vi "Get SMO PGSQL Log Paths.vi"(5 "getAll Cluster":variant, 7 "Paths":string="llab_038:d000(TEST_TABLE--Temperature(Kelvin))\nllab_038:d002(TEST_TABLE--voltage 2(volts))\nllab_038:b000(TEST_TABLE--ON?())\nllab_038:v001(TEST_TABLE--sample())", 8 "error in (no error)":errorcluster, 11 "Inst.SPC in":refnum<class "Inst.SPC.lvclass">) -> (0 "error out":errorcluster, 2 "Paths":string, 3 "Inst.SPC out":refnum<class "Inst.SPC.lvclass">)   [LabVIEW 2019, in "Inst.SPC.lvclass"]
uses:
  Inst.SPC.lvclass
  Typedefs/Inst.SPC.getAll--Cluster.ctl
  <userlib>/LevyLab/Instrument Framework/Instrument Types/VSource/Instrument.VSource.lvclass
  <userlib>/LevyLab/LV-Data/LV-Data.PG/LV-Data.PGSQL.lvclass
  <userlib>/LevyLab/LV-Data/LV-Data.PG/API/Write Variable (one-row).vi
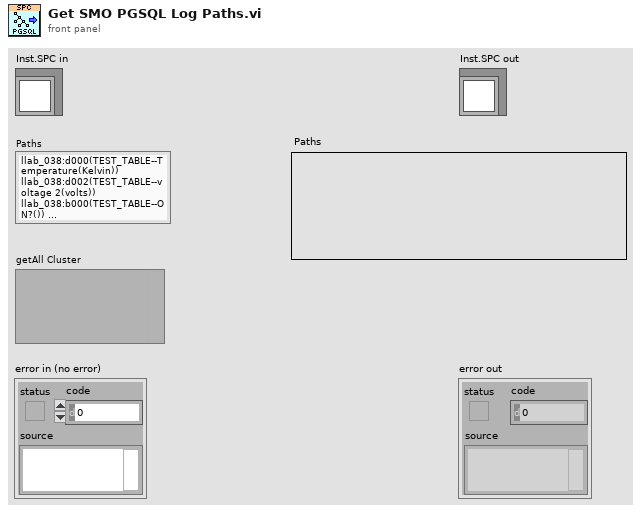
[diagram p1: front panel]
types:
  T1 = typedef "Inst.SPC.lvclass/Inst.SPC.getAll--Cluster.ctl" = cluster{"Levy 1":dbl, "Logger SMO":dbl, "SMO Boolean":bool, "SMO String":string}
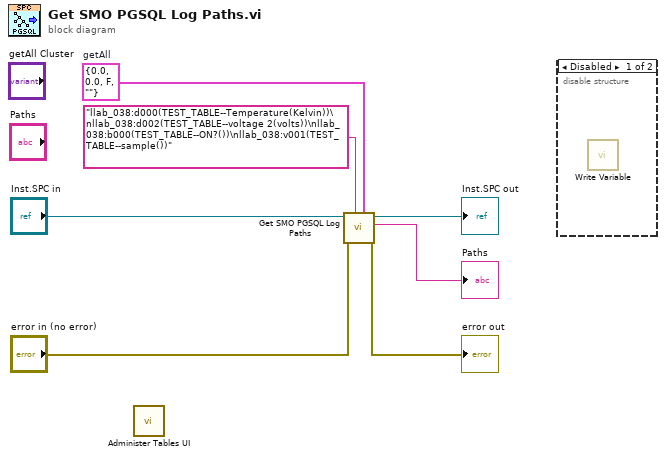
[diagram p0: block diagram]
diagram:
  w1 = T1 {"Levy 1"=0.0, "Logger SMO"=0.0, "SMO Boolean"=FALSE, "SMO String"=""}  # getAll
  n1 = call <userlib>:"Administer Tables UI.vi"() -> ()  [unwired: 12 in]
  n2 = call-parent "Get SMO PGSQL Log Paths.vi"("getAll Cluster"=w1, "Default Paths"="llab_038:d000(TEST_TABLE--Temperature(Kelvin))\nllab_038:d002(TEST_TABLE--voltage 2(volts))\nllab_038:b000(TEST_TABLE--ON?())\nllab_038:v001(TEST_TABLE--sample())" ("Paths"), "error in (no error)"="error in (no error)", "Instrument in"="Inst.SPC in") -> ("error out"=→"error out":errorcluster, "Paths"=→"Paths":string, "Instrument out"=→"Inst.SPC out":refnum<class "Inst.SPC.lvclass">)  [unwired: 5 in]
  n3 = disable-structure shown="Disabled" {
    frame Disabled {
      n4 = call-poly <userlib>:"Write Variable.vi"() -> ()  [unwired: 8 in, 4 out]
    }
    frame Enabled {
    }
  }
